vi "Read Settings.vi"(8 "error in (no error)":errorcluster, 11 "LR-700 in":refnum<class "LR-700.lvclass">) -> (0 "error out":errorcluster, 2 "Settings":string, 3 "LR-700 out":refnum<class "LR-700.lvclass">)   [LabVIEW 2015, in "LR-700.lvclass"]
uses:
  LR-700.lvclass
  Instrument/Instrument.lvclass
  Instrument with scanner/Instrument with scanner.lvclass
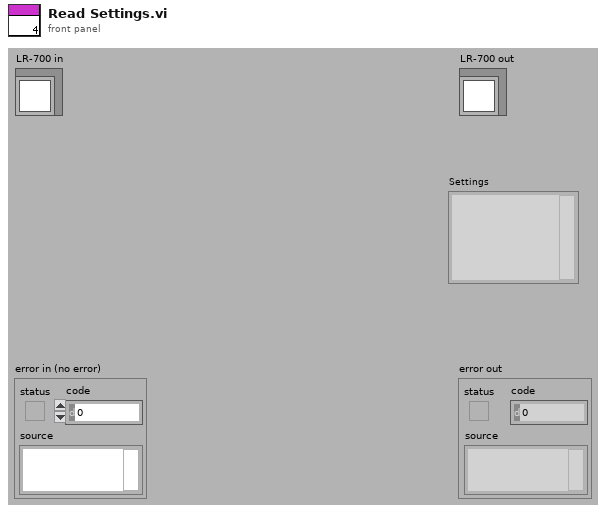
[diagram p1: front panel]
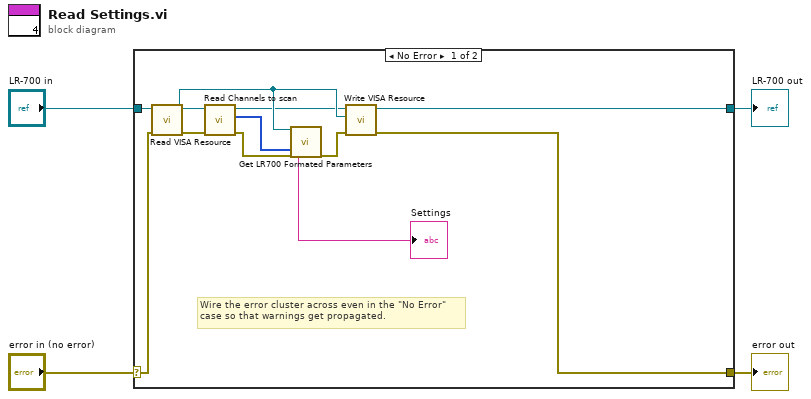
[diagram p0: block diagram]
diagram:
  n1 = case shown="No Error" "error in (no error)" {
    selector: "error in (no error)" -> [w13 w18]
    tunnel: [w11 w18] -> w3
    tunnel: [w14 w17] -> w1
    tunnel: "LR-700 in" -> [w16 w17]
    frame No Error {
      # "Wire the error cluster across even in the \"No Error\"\ncase so that warnings get propagated."
      n2 = call "Read VISA Resource.vi"("error in (no error)"=w13, "Instrument.lvclass in"=w16) -> ("error out"=w8:errorcluster, "VISA Resource"=w10:refnum<visa-resource-name>, "Instrument.lvclass out"=w15:refnum<class "LR-700.lvclass">)  [unwired: 7 out]
      n3 = call "Read Channels to scan.vi"("error in (no error)"=w8, "Instrument with scanner.lvclass in"=w15) -> ("error out"=w6:errorcluster, "Channels to scan (empty - don't use scanner option)"=w7:i32[], "Instrument with scanner.lvclass out"=w9:refnum<class "LR-700.lvclass">)  [unwired: 7 out]
      n4 = call "Get LR700 Formated Parameters.vi"("VISA Resource Name"=w10, "Channels to scan (empty - don't use scanner option)"=w7, "error in (no error)"=w6) -> ("Parameters"=→"Settings":string, "error out"=w12:errorcluster)  [unwired: 1 in, 14 out]
      n5 = call "Write VISA Resource.vi"("error in (no error)"=w12, "VISA Resource"=w10, "Instrument.lvclass in"=w9) -> ("error out"=w11:errorcluster, "Instrument.lvclass out"=w14:refnum<class "LR-700.lvclass">)  [unwired: 7 out]
    }
    frame Error {
    }
  }
  "error out" <- w3
  "LR-700 out" <- w1
